vi "读文件.vi"() -> ()   [LabVIEW 2021]
doc: "本VI是为《我和LabVIEW》一书编写的示例。\n关于本书的介绍请参考网页：\nhttp://ruanqizhen.spaces.live.com/blog/cns!5852D4F797C53FB6!4310.entry"
panel:
  out "实验数据":dbl[][](array[numeric])
  out "实验时间":timestamp
  out "实验名称":string
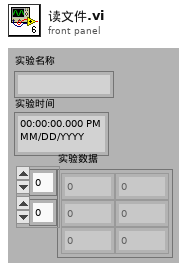
[diagram p1: front panel]
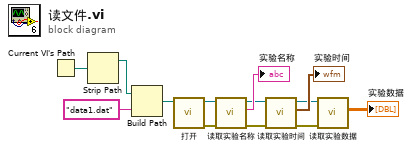
[diagram p0: block diagram]
diagram:
  n1 = Current VI's Path() -> (path=w11:path)
  n2 = Strip Path(path=w11) -> (stripped path=w12:path)  [unwired: 1 out]
  n3 = Build Path(base path=w12, name or relative path="data1.dat" ("名称或相对路径")) -> (appended path=w10:path)
  n4 = call "打开.vi"("路径"=w10) -> ("error out"=w8:errorcluster, "数据文件.lvclass"=w9:refnum<class "数据文件.lvclass">)  [unwired: 9 in]
  n5 = call-dynamic "读取实验名称.vi"("error in (no error)"=w8, "数据文件.lvclass"=w9) -> ("error out"=w5:errorcluster, "实验名称"=→"实验名称":string, "数据文件.lvclass"=w6:refnum<class "数据文件.lvclass">)  [unwired: 7 in]
  n6 = call-dynamic "读取实验时间.vi"("error in (no error)"=w5, "数据文件.lvclass"=w6) -> ("error out"=w2:errorcluster, "实验时间"=→"实验时间":timestamp, "数据文件.lvclass"=w3:refnum<class "数据文件.lvclass">)  [unwired: 7 in]
  n7 = call-dynamic "读取实验数据.vi"("error in (no error)"=w2, "数据文件.lvclass"=w3) -> ("实验数据"=→"实验数据":dbl[][])  [unwired: 7 in, 2 out]
